vi "GetEnvCover.vi"(7 "LabVIEW Web Service Request":refnum<class "Web Request.lvclass">) -> (3 "EnvCover":string)   [LabVIEW 2016]
uses:
  <vilib>/wsapi/Web Request.lvclass
  controls/MotorStates.ctl
panel:
  # "Use the Web Service Request input terminal to call the VIs on the Web Services palette. Do not remove it from the connector pane unless you don't need access to the palette."
  # "Each additional control wired to the connector pane will be available as an input in the URL. To include an indicator in terminal-mode output (the default setting), it must also be wired to the connector pane."
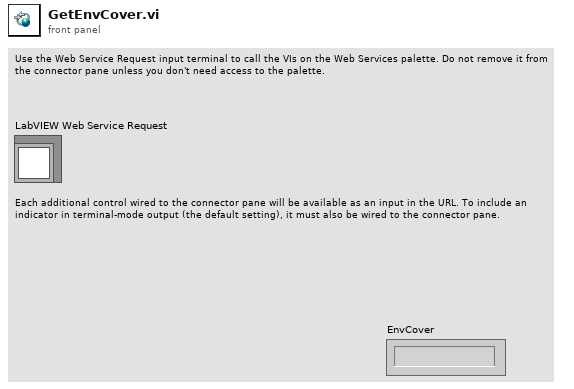
[diagram p1: front panel]
types:
  T1 = typedef "RT-Variables.lvlib/MotorStates.ctl" = enum16{"Open", "Close", "Moving"}
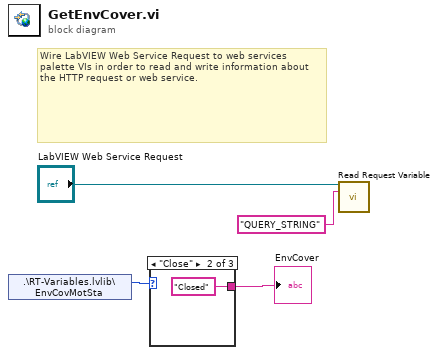
[diagram p0: block diagram]
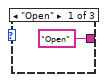
[diagram p2: hidden frame]
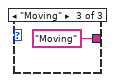
[diagram p3: hidden frame]
diagram:
  # "Wire LabVIEW Web Service Request to web services palette VIs in order to read and write information about the HTTP request or web service."
  n1 = shared-variable ".\\RT-Variables.lvlib\\EnvCovMotSta"() -> (w1:T1)  [unwired: 1 in, 1 out]
  n2 = case shown="\"Close\"" w1 {
    tunnel: ["Open" ("EnvCover") "Closed" ("EnvCover") "Moving" ("EnvCover")] -> w2
    frame "Open" {
    }
    frame "Close" {
    }
    frame "Moving" {
    }
  }
  "EnvCover" <- w2
  n3 = call <vilib>:"Read Request Variable.vi"("LabVIEW Web Service Request"="LabVIEW Web Service Request", "variable name"="QUERY_STRING") -> ()  [unwired: 11 in, 3 out]
